vi "filter test.vi"() -> ()   [LabVIEW 2016]
uses:
  viz_filter options.ctl
  viz_filter.ctl
  viz_entry.ctl
  <vilib>/NI Veristand/Custom Device API/Custom Device Item Ref.ctl
  Client/Test CD/FPGA RM Test Client/Source/System Explorer/Filters/Filter Parent/Filter.lvclass
  RM.Server.lvlib
  <vilib>/NI VeriStand/Custom Device API/Custom Device API.lvlib
panel:
  out "resource entries out":T1[](array[typedef]) {"FPGA CD Ref" format="%.0x"; "reserver" format="%.0x"}
  in  "resource entries in":T1[](array[typedef]) {"FPGA CD Ref" format="%.0x"; "reserver" format="%.0x"}
  in  "Filters":T3[](array[typedef])
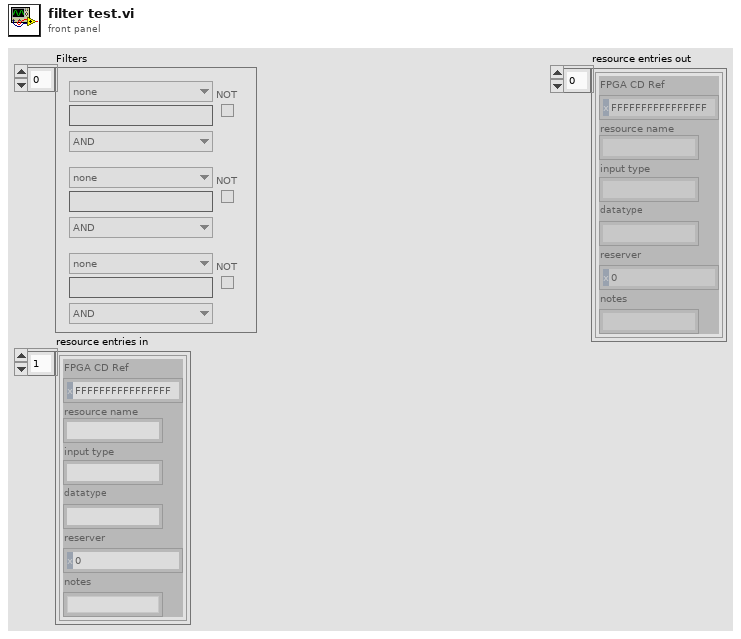
[diagram p1: front panel]
types:
  T1 = typedef "RM.Server.lvlib/viz_entry.ctl" = cluster{"FPGA CD Ref":T2, "resource name":string, "input type":string, "datatype":string, "reserver":T2, "notes":string}
  T2 = typedef "Custom Device API.lvlib/Custom Device Item Ref.ctl" = u64
  T3 = typedef "RM.Server.lvlib/viz_filter options.ctl" = cluster{"Filter Options":cluster{"Filter Type":T4, "Filter Value":string, "NOT":bool}, "next filter boolean":enum16{"AND", "OR"}}
  T4 = typedef "RM.Server.lvlib/viz_filter.ctl" = enum16{"none", "RIO Device", "Resource Name", "Input Type", "Datatype"}
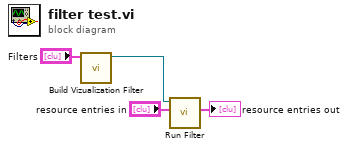
[diagram p0: block diagram]
diagram:
  n1 = call "Build Vizualization Filter.vi"("Filters"="Filters") -> ("Filter out"=w3:refnum<class "Filter.lvclass">)  [unwired: 10 in]
  n2 = call-dynamic "Run Filter.vi"("resource entries in"="resource entries in", "Filter in"=w3) -> ("resource entries out"=→"resource entries out":T1[])  [unwired: 8 in, 1 out]
